vi "DB Tools Open Schema.vi"(4 "column":i32, 5 "error in (no error)":errorcluster, 6 "constraint information":T1, 7 "Schema":i32(ring)=-1 items=["adSchemaProviderSpecific"=-1, "adSchemaAsserts"=0, "adSchemaCatalogs"=1, "adSchemaCharacterSets"=2, "adSchemaCollations"=3, "adSchemaColumns"=4, "adSchemaCheckConstraints"=5, "adSchemaConstraintColumnUsage"=6, "adSchemaConstraintTableUsage"=7, "adSchemaKeyColumnUsage"=8, "adSchemaReferentialContraints, adSchemaReferentialConstraints"=9, "adSchemaTableConstraints"=10, "adSchemaColumnsDomainUsage"=11, "adSchemaIndexes"=12, "adSchemaColumnPrivileges"=13, "adSchemaTablePrivileges"=14, "adSchemaUsagePrivileges"=15, "adSchemaProcedures"=16, "adSchemaSchemata"=17, "adSchemaSQLLanguages"=18, "adSchemaStatistics"=19, "adSchemaTables"=20, "adSchemaTranslations"=21, "adSchemaProviderTypes"=22, "adSchemaViews"=23, "adSchemaViewColumnUsage"=24, "adSchemaViewTableUsage"=25, "adSchemaProcedureParameters"=26, "adSchemaForeignKeys"=27, "adSchemaPrimaryKeys"=28, "adSchemaProcedureColumns"=29, "adSchemaDBInfoKeywords"=30, "adSchemaDBInfoLiterals"=31, "adSchemaCubes"=32, "adSchemaDimensions"=33, "adSchemaHierarchies"=34, "adSchemaLevels"=35, "adSchemaMeasures"=36, "adSchemaProperties"=37, "adSchemaMembers"=38, "adSchemaTrustees"=39], 8 "connection reference":T2) -> (0 "error out":errorcluster, 2 "schema data":string[](array[string]), 3 "connection reference out":T2)   [LabVIEW 2017, in "NI_Database_API.lvlib"]
doc: "Returns information about the data source defined by the <B>connection reference</B>, such as information about the tables on the server and the columns in the tables. The <B>schema</B> input specifies the type of schema query to run. \n\nThe <B>constraint information</B> is a cluster of values that limit the results of a schema query. Each schema query has a different set of parameters that it supports. The actual schemas are defined by the OLE DB specification. \n\nNote: Providers are not required to support all of the OLE DB standard schema queries. Specifically, only adSchemaTables, adSchemaColumns, and adSchemaProviderTypes are required by the OLE DB specification. However, the provider is not required to support the constraint information for those schema queries."
uses:
  <vilib>/addons/database/NI_Database_API.lvlib
  <vilib>/addons/database/Connection.llb/Conn ObjectReference.ctl
  <vilib>/addons/database/Auxilliary.llb/DB Tools Constraint Info.ctl
  <vilib>/addons/database/_DB Variant To Data/Database Variant To Data.xnode
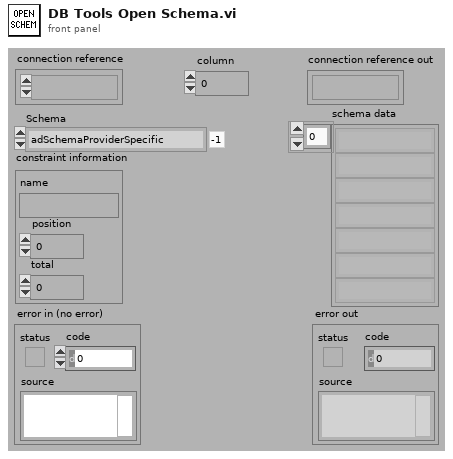
[diagram p1: front panel]
types:
  T1 = typedef "NI_Database_API.lvlib/DB Tools Constraint Info.ctl" = cluster{"name":string, "position":i32, "total":i32}
  T2 = typedef "NI_Database_API.lvlib/Conn ObjectReference.ctl" = refnum<k1>
  T3 = typedef "NI_Database_API.lvlib/Conn DataMembers.ctl" = cluster{"ADODB._Connection":refnum<k7>, "recordset objects":i32, "command objects":i32}
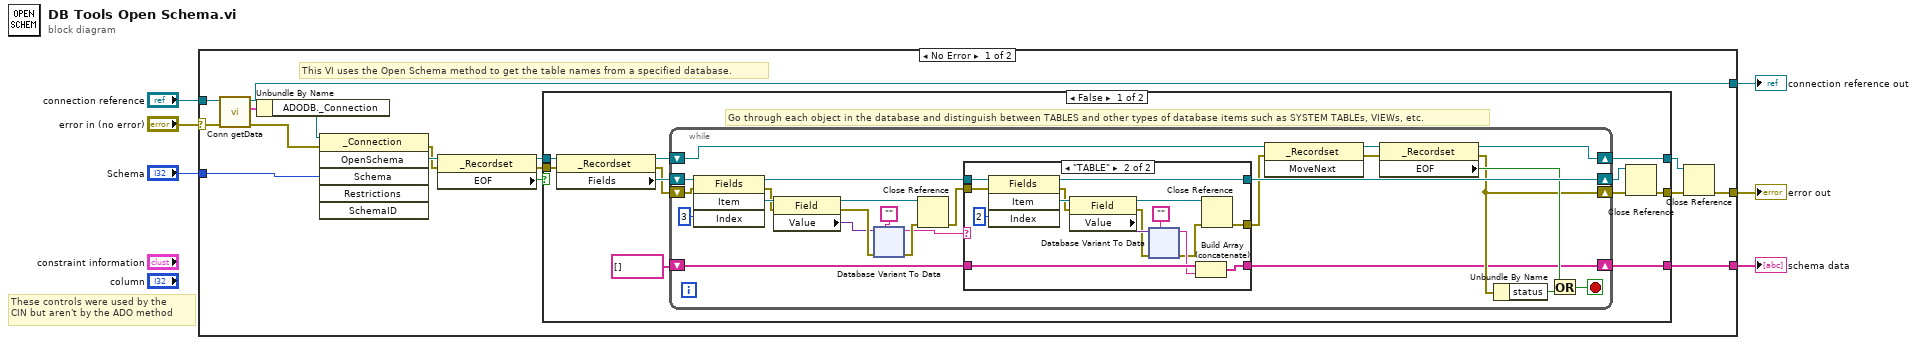
[diagram p0: block diagram]
diagram:
  # "These controls were used by the \nCIN but aren't by the ADO method"
  n1 = case shown="No Error" "error in (no error)" {
    selector: "error in (no error)" -> [w7 w144]
    tunnel: "connection reference" -> [w21 w143]
    tunnel: "Schema" -> [w19 _]
    tunnel: [w17 w143] -> w4
    tunnel: [w16 _] -> w3
    tunnel: [w14 w144] -> w2
    frame No Error {
      # "This VI uses the Open Schema method to get the table names from a specified database."
      n2 = call <vilib>:"Conn getData.vi"("error in (no error)"=w7, "connection reference"=w21) -> ("error out"=w18:errorcluster, "data"=w22:T3, "connection reference out"=w17:T2)  [unwired: 2 in, 1 out]
      n3 = Unbundle By Name(w22) -> ("ADODB._Connection"=w20:refnum<k7>)
      n4 = invoke class="_Connection" method="OpenSchema"(reference=w20, error in=w18, "Schema"=w19) -> (error out=w10:errorcluster, "OpenSchema"=w12:refnum<k7>)  [unwired: 3 in, 4 out]
      n5 = property class="_Recordset"(reference=w12, error in=w10) -> (reference out=w11:refnum<k7>, error out=w9:errorcluster, "EOF"=w8:bool)
      n6 = case shown="False" w8 {
        tunnel: [w30 _] -> w16
        tunnel: [w27 w141] -> w15
        tunnel: [w25 w142] -> w13
        tunnel: w11 -> [w24 w142]
        tunnel: w9 -> [w23 w141]
        frame False {
          # "Go through each object in the database and distinguish between TABLES and other types of database items such as SYSTEM TABLEs, VIEWs, etc."
          n7 = property class="_Recordset"(reference=w24, error in=w23) -> (reference out=w33:refnum<k7>, error out=w31:errorcluster, "Fields"=w32:refnum<k7>)
          n8 = while {
            shift-right: [w50] -> w26
            shift-left: w32 -> [w58]
            shift-right: [w44] -> w28
            shift-left: w31 -> [w56]
            shift-right: [w53] -> w25
            shift-left: w33 -> [w35]
            shift-right: [w41] -> w30
            shift-left: string[] [] -> [w42]
            stop <- w57 stop-if-true
            n9 = invoke class="Fields" method="Item"(reference=w58, error in=w56, "Index"=3) -> (reference out=w51:refnum<k7>, error out=w34:errorcluster, "Item"=w49:refnum<k7>)  [unwired: 1 in, 1 out]
            n10 = property class="Field"(reference=w49, error in=w34) -> (reference out=w39:refnum<k7>, error out=w47:errorcluster, "Value"=w40:variant)
            n11 = xnode "Database Variant To Data"("database variant"=w40, "error in"=w47, "type"="") -> ("data"=w36:string, "error out"=w38:errorcluster)
            n12 = Close Reference(reference=w39, error in (no error)=w38) -> (error out=w37:errorcluster)
            n13 = case shown="\"TABLE\"" w36 {
              tunnel: [w92 w101] -> w41
              tunnel: w51 -> [w93 w107]
              tunnel: [w93 w105] -> w50
              tunnel: [w91 w95] -> w43
              tunnel: w42 -> [w92 w102]
              tunnel: w37 -> [w91 w97]
              frame Default {
              }
              frame "TABLE" {
                n14 = invoke class="Fields" method="Item"(reference=w107, error in=w97, "Index"=2) -> (reference out=w105:refnum<k7>, error out=w104:errorcluster, "Item"=w106:refnum<k7>)  [unwired: 1 in, 1 out]
                n15 = property class="Field"(reference=w106, error in=w104) -> (reference out=w94:refnum<k7>, error out=w98:errorcluster, "Value"=w99:variant)
                n16 = xnode "Database Variant To Data"("database variant"=w99, "error in"=w98, "type"="") -> ("data"=w100:string, "error out"=w96:errorcluster)
                n17 = Build Array (concatenate)(w102, w100) -> (w101:string[])
                n18 = Close Reference(reference=w94, error in (no error)=w96) -> (error out=w95:errorcluster)
              }
            }
            n19 = invoke class="_Recordset" method="MoveNext"(reference=w35, error in=w43) -> (reference out=w55:refnum<k7>, error out=w54:errorcluster)  [unwired: 1 in, 1 out]
            n20 = property class="_Recordset"(reference=w55, error in=w54) -> (reference out=w53:refnum<k7>, error out=w44:errorcluster, "EOF"=w45:bool)
            n21 = Unbundle By Name(w44) -> ("status"=w52:bool)
            n22 = Or(x=w45, y=w52) -> (x .or. y?=w57:bool)
          }
          n23 = Close Reference(reference=w26, error in (no error)=w28) -> (error out=w27:errorcluster)
        }
        frame True {
          # "No objects in the database."
        }
      }
      n24 = Close Reference(reference=w13, error in (no error)=w15) -> (error out=w14:errorcluster)
    }
    frame Error {
    }
  }
  "connection reference out" <- w4
  "error out" <- w2
  "schema data" <- w3
